vi "set_FPGA_VI_ref.vi"(8 "error in (no error)":errorcluster, 10 "FPGA VI reference":T1, 11 "FPGAWrapperAN110607Galvo in":refnum<class "FPGAWrapperAN110607Galvo.lvclass">) -> (0 "error out":errorcluster, 3 "FPGAWrapperAN110607Galvo out":refnum<class "FPGAWrapperAN110607Galvo.lvclass">)   [LabVIEW 2010, in "FPGAWrapperAN110607Galvo.lvclass"]
uses:
  FPGAWrapperAN110607Galvo.lvclass
  FPGA_VI_ref.ctl
  class_data.vi
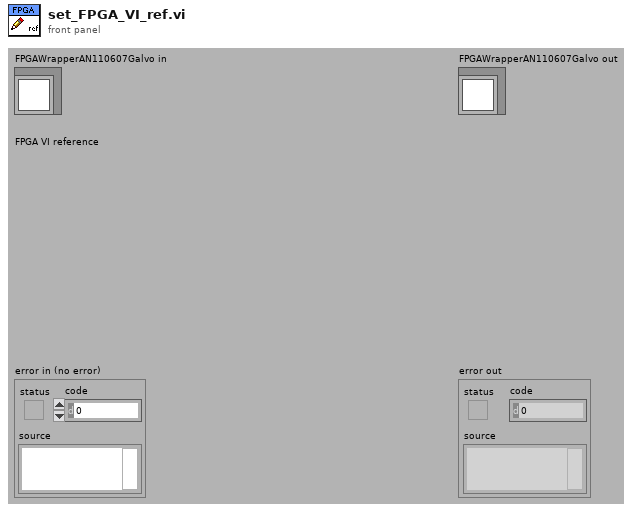
[diagram p1: front panel]
types:
  T1 = typedef "FPGAWrapperAN110607Galvo.lvclass/FPGA_VI_ref.ctl" = refnum<k20>
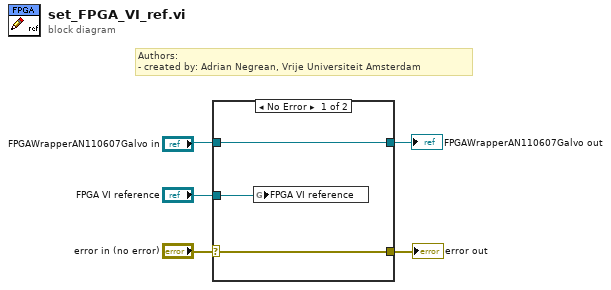
[diagram p0: block diagram]
diagram:
  # "Authors: \n- created by: Adrian Negrean, Vrije Universiteit Amsterdam"
  n1 = case shown="No Error" "error in (no error)" {
    selector: "error in (no error)" -> [w7 w10]
    tunnel: [w7 w10] -> w4
    tunnel: [w8 w9] -> w2
    tunnel: "FPGAWrapperAN110607Galvo in" -> [w8 w9]
    tunnel: "FPGA VI reference" -> [w6 _]
    frame No Error {
      n2 = global write "class_data.vi" "FPGA VI reference"(w6) -> ()
    }
    frame Error {
    }
  }
  "error out" <- w4
  "FPGAWrapperAN110607Galvo out" <- w2
